vi "model debug.vi"() -> ()   [LabVIEW 2022 SP3]
uses:
  Model/Serial port assistant model.lvclass
panel:
  in  "DATA":string
  in  "Clear":bool
  in  "Exit":bool
  out "changed data":string
  out "view number":i32
  out "view name":string
  in  "close serial port":bool
  in  "stop receiving data":bool
  in  "send data":bool
  in  "start receiving data":bool
  in  "open serial port":bool
  in  "query serial port list":bool
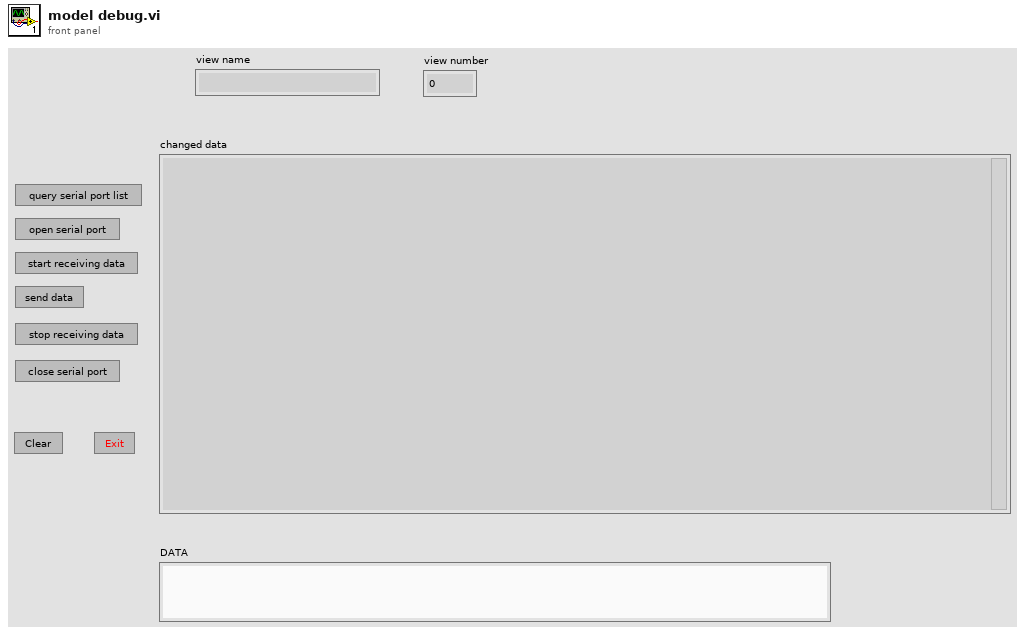
[diagram p1: front panel]
types:
  T1 = cluster{"request":string, "data to be sent":string}
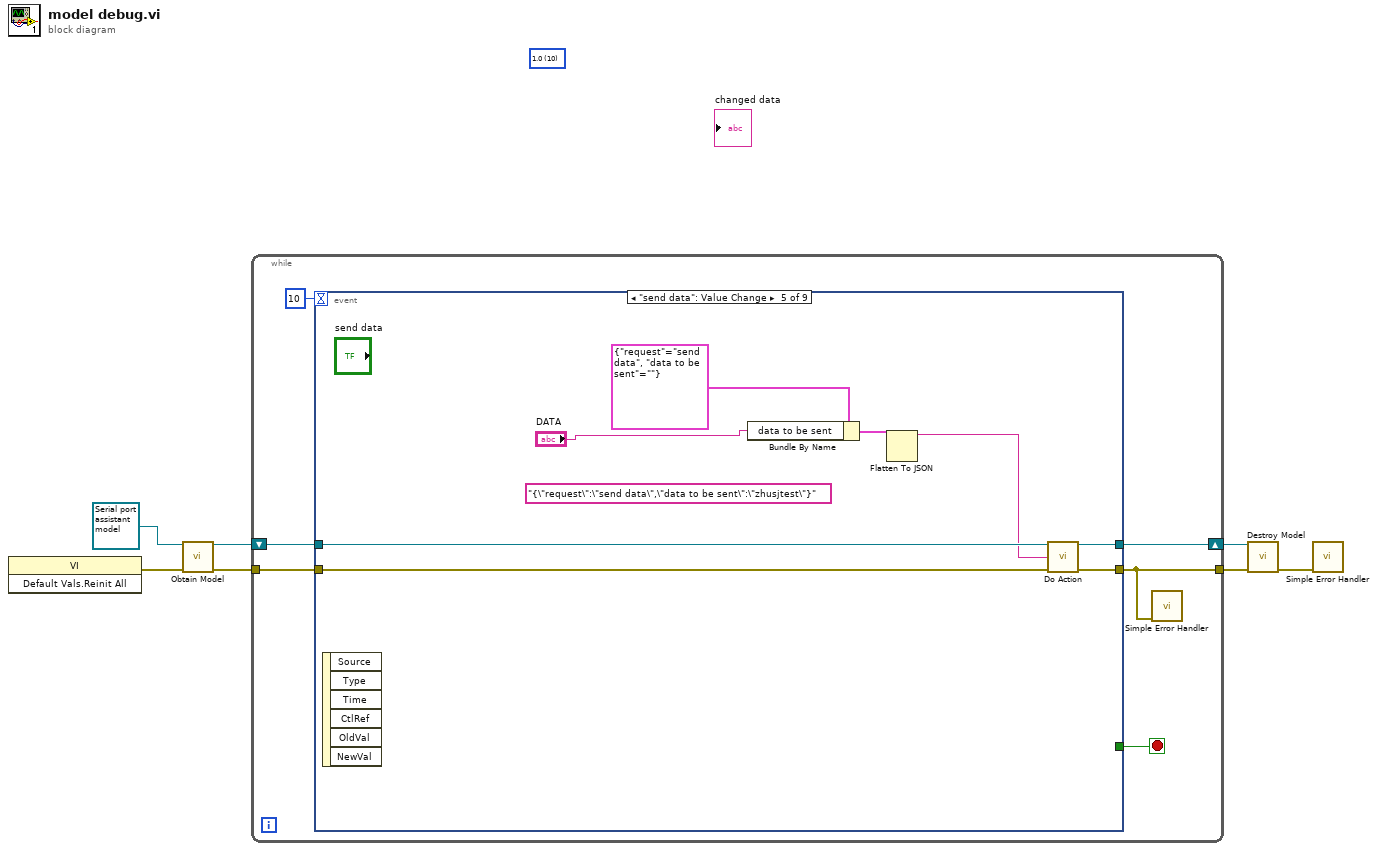
[diagram p0: block diagram]
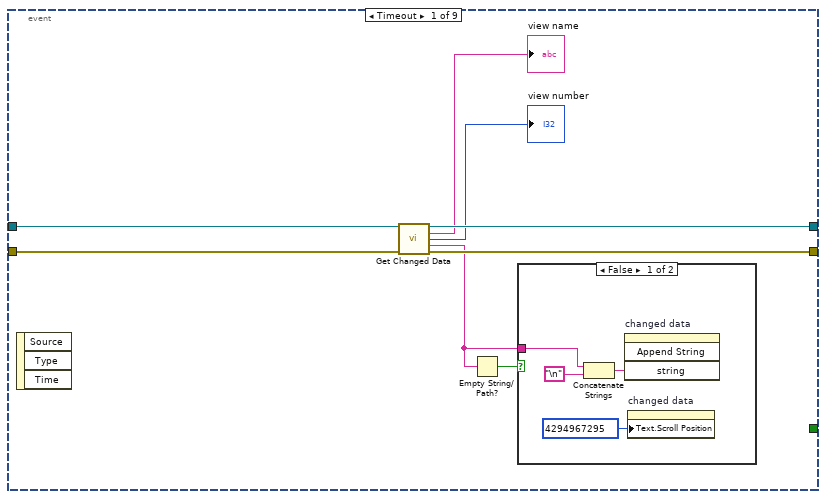
[diagram p2: hidden frame]
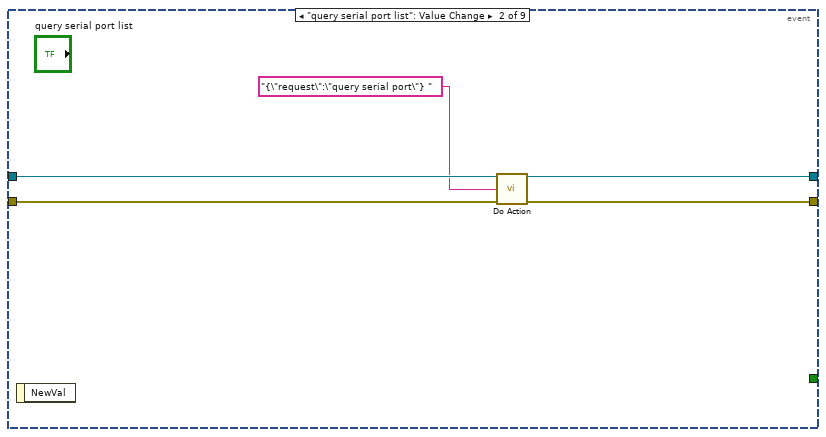
[diagram p4: hidden frame]
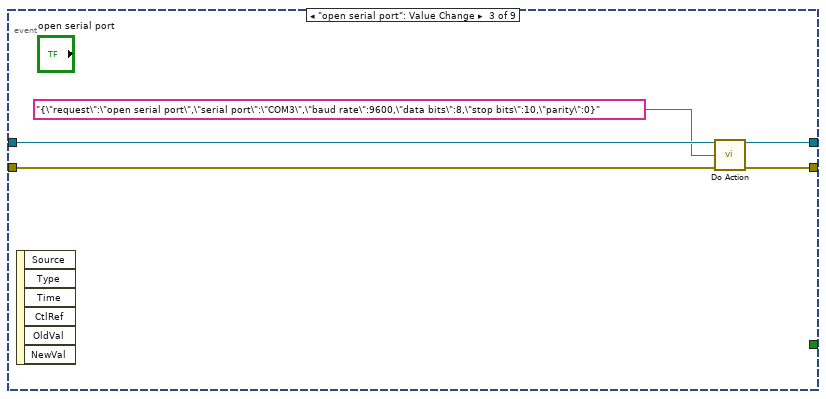
[diagram p5: hidden frame]
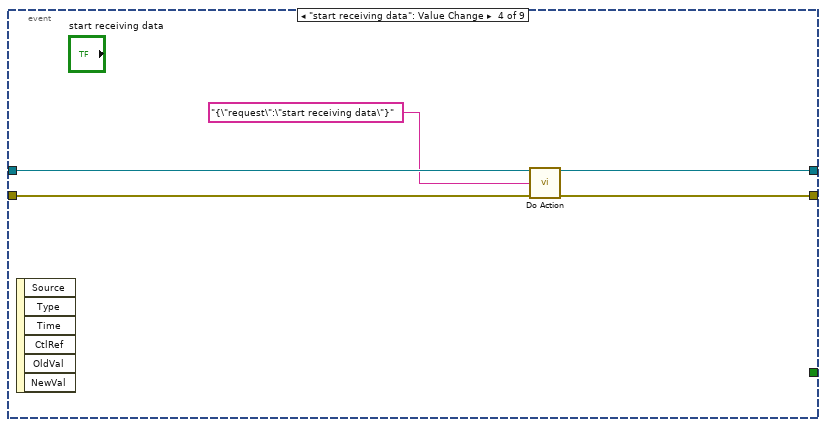
[diagram p6: hidden frame]
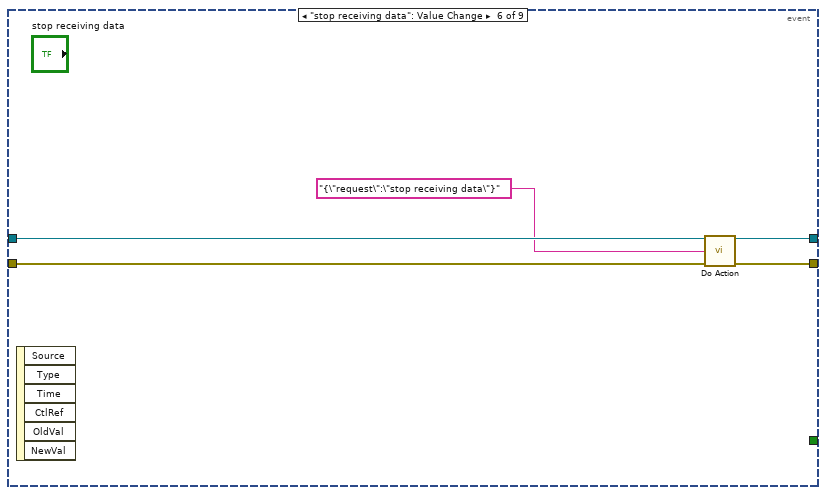
[diagram p7: hidden frame]
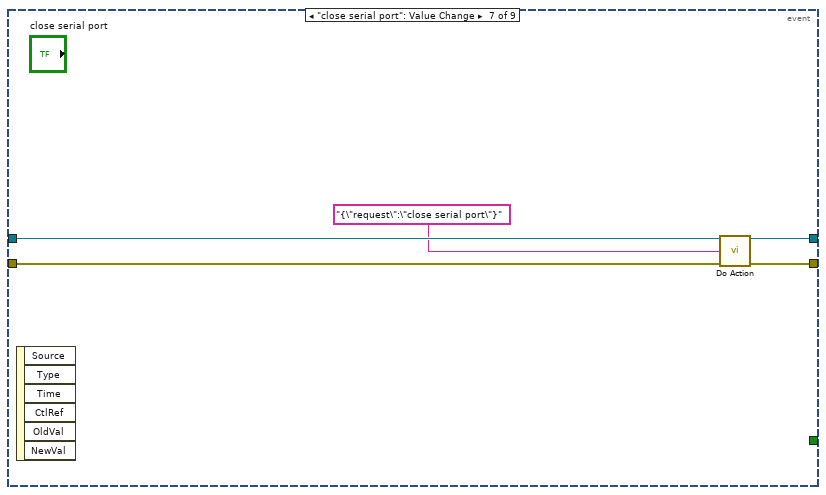
[diagram p8: hidden frame]
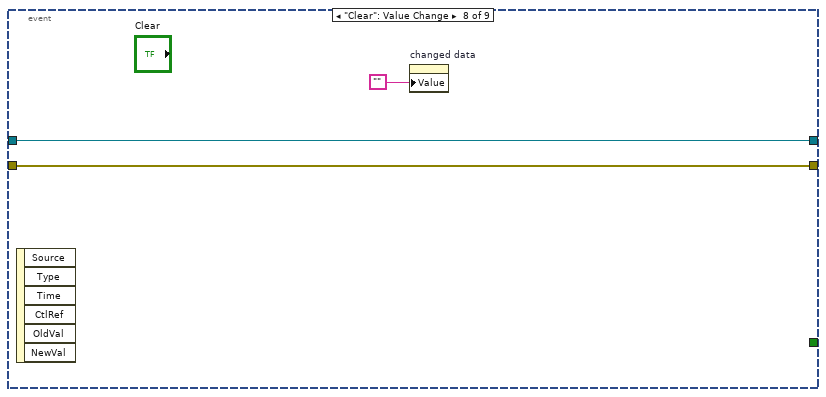
[diagram p9: hidden frame]
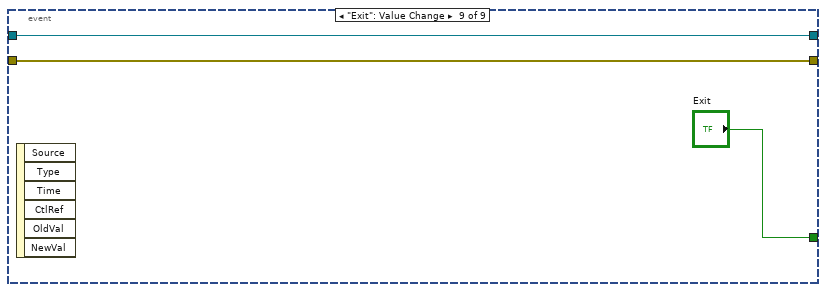
[diagram p10: hidden frame]
diagram:
  (unwired) u16 10 items=["1.0"=10, "1.5"=15, "2.0"=20] ("stop bits (10: 1 bit)")
  n1 = invoke class="VI" method="Default Vals.Reinit All"() -> (error out=w2:errorcluster)  [unwired: 3 in, 2 out]
  n2 = call-dynamic "Obtain Model.vi"("Serial port asssistant model in"=refnum<class "Serial port assistant model.lvclass"> refnum, "error in (no error)"=w2) -> ("Serial port asssistant model out"=w6:refnum<class "Serial port assistant model.lvclass">, "error out"=w5:errorcluster)  [unwired: 12 in]
  n3 = while {
    shift-right: [w10] -> w3
    shift-left: w6 -> [w12]
    tunnel: w5 -> [w13]
    tunnel: [w8] -> w4
    stop <- w9 stop-if-true
    n4 = event shown="[4] \"send data\": Value Change" {
      selector: _ -> [_ _ _ _ _ _ _ _ _]
      dyn-events: _ -> [_ _ _ _ _ _ _ _ _]
      timeout: 10 -> [_ _ _ _ _ _ _ _ _]
      tunnel: w13 -> [w21 w28 w34 w39 w48 w53 w58 w61 w64]
      tunnel: w12 -> [w20 w30 w35 w40 w47 w52 w57 w60 w63]
      tunnel: [w19 w29 w33 w37 w46 w50 w56 w60 w63] -> w10
      tunnel: [w18 w27 w32 w38 w45 w51 w55 w61 w64] -> w8
      tunnel: [_ _ _ _ _ _ _ _ "Exit"] -> w9
      event Timeout {
        n5 = event-data() -> ()  [unwired: 1 in, 3 out]
        n6 = call-dynamic "Get Changed Data.vi"("Serial port asssistant model in"=w20, "error in (no error)"=w21) -> ("Serial port asssistant model out"=w19:refnum<class "Serial port assistant model.lvclass">, "view name"=→"view name":string, "view number"=→"view number":i32, "changed data"=w14:string, "error out"=w18:errorcluster)  [unwired: 9 in]
        n7 = Empty String/Path?(string/path=w14) -> (empty?=w15:bool)
        n8 = case shown="False" w15 {
          tunnel: w14 -> [w23 _]
          frame False {
            n9 = Concatenate Strings(w23, "\n") -> (w25:string)
            n10 = invoke on="changed data" class="Str" method="Append String"("string"=w25) -> ()  [unwired: 3 in, 4 out]
            n11 = property on="changed data" class="Str"("Text.Scroll Position"=u32 4294967295) -> ()  [unwired: 2 in, 2 out]
          }
          frame True {
          }
        }
      }
      event "query serial port list": Value Change {
        n12 = event-data() -> ()  [unwired: 1 in, 1 out]
        n13 = call-dynamic "Do Action.vi"("Serial port asssistant model in"=w30, "request"="{\"request\":\"query serial port\"} ", "error in (no error)"=w28) -> ("Serial port asssistant model out"=w29:refnum<class "Serial port assistant model.lvclass">, "error out"=w27:errorcluster)  [unwired: 11 in]
      }
      event "open serial port": Value Change {
        n14 = event-data() -> ()  [unwired: 1 in, 6 out]
        n15 = call-dynamic "Do Action.vi"("Serial port asssistant model in"=w35, "request"="{\"request\":\"open serial port\",\"serial port\":\"COM3\",\"baud rate\":9600,\"data bits\":8,\"stop bits\":10,\"parity\":0}", "error in (no error)"=w34) -> ("Serial port asssistant model out"=w33:refnum<class "Serial port assistant model.lvclass">, "error out"=w32:errorcluster)  [unwired: 11 in]
      }
      event "start receiving data": Value Change {
        n16 = event-data() -> ()  [unwired: 1 in, 6 out]
        n17 = call-dynamic "Do Action.vi"("Serial port asssistant model in"=w40, "request"="{\"request\":\"start receiving data\"}", "error in (no error)"=w39) -> ("Serial port asssistant model out"=w37:refnum<class "Serial port assistant model.lvclass">, "error out"=w38:errorcluster)  [unwired: 11 in]
      }
      event "send data": Value Change {
        (unwired) "{\"request\":\"send data\",\"data to be sent\":\"zhusjtest\"}" ("request")
        n18 = event-data() -> ()  [unwired: 1 in, 6 out]
        n19 = Bundle By Name(cluster=T1 {"request"="send data", "data to be sent"=""}, "data to be sent"="DATA") -> (w42:T1)
        n20 = Flatten To JSON(anything=w42) -> (JSON string=w41:string)  [unwired: 2 in, 1 out]
        n21 = call-dynamic "Do Action.vi"("Serial port asssistant model in"=w47, "request"=w41, "error in (no error)"=w48) -> ("Serial port asssistant model out"=w46:refnum<class "Serial port assistant model.lvclass">, "error out"=w45:errorcluster)  [unwired: 11 in]
      }
      event "stop receiving data": Value Change {
        n22 = event-data() -> ()  [unwired: 1 in, 6 out]
        n23 = call-dynamic "Do Action.vi"("Serial port asssistant model in"=w52, "request"="{\"request\":\"stop receiving data\"}", "error in (no error)"=w53) -> ("Serial port asssistant model out"=w50:refnum<class "Serial port assistant model.lvclass">, "error out"=w51:errorcluster)  [unwired: 11 in]
      }
      event "close serial port": Value Change {
        n24 = event-data() -> ()  [unwired: 1 in, 6 out]
        n25 = call-dynamic "Do Action.vi"("Serial port asssistant model in"=w57, "request"="{\"request\":\"close serial port\"}", "error in (no error)"=w58) -> ("Serial port asssistant model out"=w56:refnum<class "Serial port assistant model.lvclass">, "error out"=w55:errorcluster)  [unwired: 11 in]
      }
      event "Clear": Value Change {
        n26 = event-data() -> ()  [unwired: 1 in, 6 out]
        n27 = property on="changed data" class="Str"("Value"="") -> ()  [unwired: 2 in, 2 out]
      }
      event "Exit": Value Change {
        n28 = event-data() -> ()  [unwired: 1 in, 6 out]
      }
    }
    n29 = call <vilib>:"Simple Error Handler.vi"("error in (no error)"=w8) -> ()  [unwired: 4 in, 5 out]
  }
  n30 = call-dynamic "Destroy Model.vi"("Serial port asssistant model in"=w3, "error in (no error)"=w4) -> ("error out"=w1:errorcluster)  [unwired: 12 in, 1 out]
  n31 = call <vilib>:"Simple Error Handler.vi"("error in (no error)"=w1) -> ()  [unwired: 4 in, 5 out]
